vi "Untitled 5.vi"(8 "error in (no error)":errorcluster, 11 "Autofocus in":refnum<class "Autofocus.lvclass">) -> (0 "error out":errorcluster, 3 "Autofocus out":refnum<class "Autofocus.lvclass">)   [LabVIEW 2012, in "Autofocus.lvclass"]
uses:
  Autofocus.lvclass
  Autofocus.lvclass/Autofocus.ctl
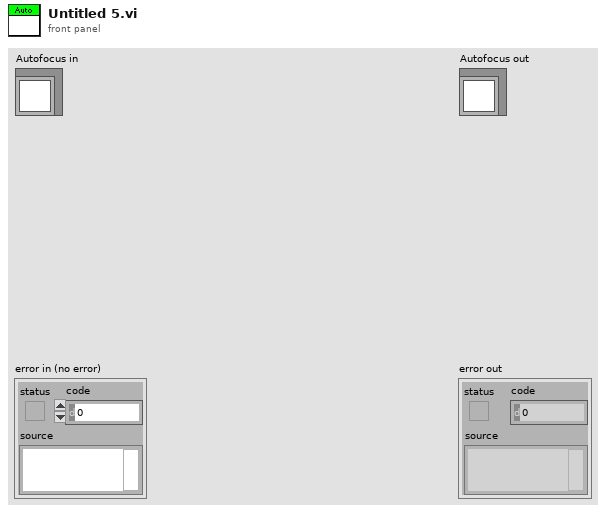
[diagram p1: front panel]
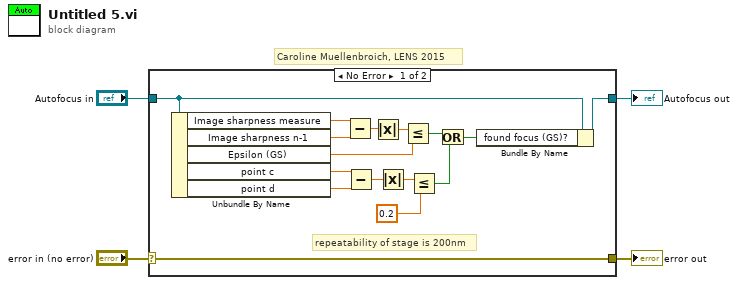
[diagram p0: block diagram]
diagram:
  # "Caroline Muellenbroich, LENS 2015"
  n1 = case shown="No Error" "error in (no error)" {
    selector: "error in (no error)" -> [w20 w22]
    tunnel: [w20 w22] -> w3
    tunnel: [w6 w21] -> w1
    tunnel: "Autofocus in" -> [w7 w21]
    frame No Error {
      # "repeatability of stage is 200nm"
      n2 = Unbundle By Name(w7) -> ("Image sharpness measure"=w19:dbl, "Image sharpness n-1"=w18:dbl, "Epsilon (GS)"=w17:dbl, "point c"=w15:dbl, "point d"=w14:dbl)
      n3 = Subtract(x=w19, y=w18) -> (x-y=w13:dbl)
      n4 = Subtract(x=w15, y=w14) -> (x-y=w11:dbl)
      n5 = Absolute Value(x=w13) -> (abs(x)=w12:dbl)
      n6 = Absolute Value(x=w11) -> (abs(x)=w10:dbl)
      n7 = Less Or Equal?(x=w12, y=w17) -> (x <= y?=w16:bool)
      n8 = Less Or Equal?(x=w10, y=0.2) -> (x <= y?=w8:bool)
      n9 = Or(x=w16, y=w8) -> (x .or. y?=w5:bool)
      n10 = Bundle By Name(cluster=w7, "found focus (GS)?"=w5) -> (w6:refnum<class "Autofocus.lvclass">)
    }
    frame Error {
    }
  }
  "error out" <- w3
  "Autofocus out" <- w1
